vi "Destroy Suite.vi"(8 "error in":errorcluster, 11 "Platano":refnum<class "Platano.CarayaTestSuite.lvclass">) -> (0 "error out":errorcluster, 3 "Test Suite Results":refnum<class "Test Result.lvclass">)   [LabVIEW 2021, in "Banana.Caraya.lvlib" / "Platano.CarayaTestSuite.lvclass"]
uses:
  Platano.CarayaTestSuite.lvclass
  C:/Repositories/LVOS/Bananas/lv-src/Bananas/Platano/Platano.lvclass
  <vilib>/addons/_JKI Toolkits/Caraya/classes/Test Result/Test Result.lvclass
  Bananas/Banana Core Actions -- enum.ctl
  Platano.CarayaTestSuite.lvclass/Platano.CarayaTestSuite.ctl
  Bananas/Banana/Banana.lvclass/Banana.ctl
  <vilib>/LabVIEW Open Source Project/Data Manipulation/Variant/Variant_SetName.vi
  <vilib>/LabVIEW Open Source Project/Data Manipulation/Variant/Variant_BuildClusterFromElementArray.vi
  Bananas/Banana/Read Ephemerals.vi
  <vilib>/LabVIEW Open Source Project/Data Manipulation/Variant/Variant_EmptyCluster.vi
  Leaf.Properties.Suite/Leaf.Properties.Suite.lvclass
  C:/Repositories/LVOS/Bananas/lv-src/Bananas/Leaf.TestSuite/Leaf.TestSuite.lvclass
  Bananas/DestroySuite/DestroySuite.lvclass
  C:/Repositories/LVOS/Bananas/lv-src/Bananas/BananaPeel/BananaPeel.lvclass
  Pips.TestResults/Pips.TestResults.lvclass
  C:/Repositories/LVOS/Bananas/lv-src/Bananas/Pips/Pips.lvclass
  <vilib>/LabVIEW Open Source Project/Data Manipulation/Variant/Variant_ListElements.vi
  <vilib>/LabVIEW Open Source Project/Data Manipulation/TypeDescriptor/TypeDescriptor_SetName.vi
  <vilib>/Utility/GetType.llb/TD_Create Cluster.vi
  Bananas/DefineTest/DefineTest.lvclass
  Bananas/DefineSuite/DefineSuite.lvclass
  Bananas/BananaPeel/BananaPeel.lvclass
  <vilib>/addons/_JKI Toolkits/Caraya/classes/Test Suite/Test Suite.lvclass
  Bananas/Banana/Banana.lvclass
  Bananas/Platano/Platano.lvclass
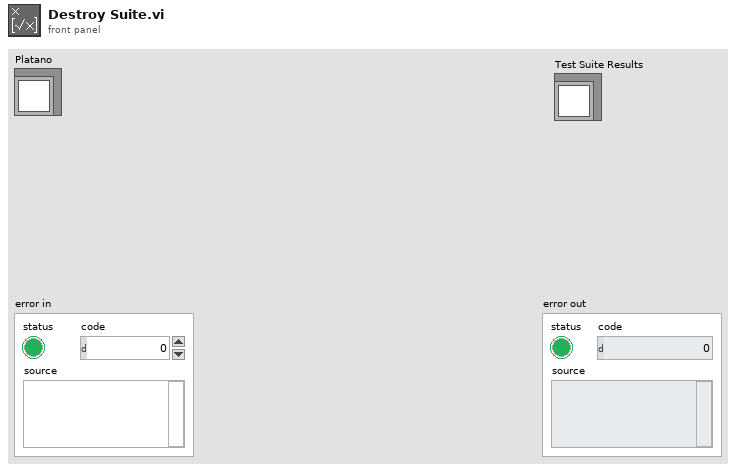
[diagram p1: front panel]
types:
  T1 = typedef "Bananas.lvlib/Banana.lvclass/Banana Core Actions -- enum.ctl" = enum16{"Get/Set", "Clear", "Discard"}
  T2 = typedef "Bananas.lvlib/Test Strategies -- cluster.ctl" = cluster{"DefineTest":refnum<class "DefineTest.lvclass">, "DefineSuite":refnum<class "DefineSuite.lvclass">, "DestroySuite":refnum<class "DestroySuite.lvclass">}
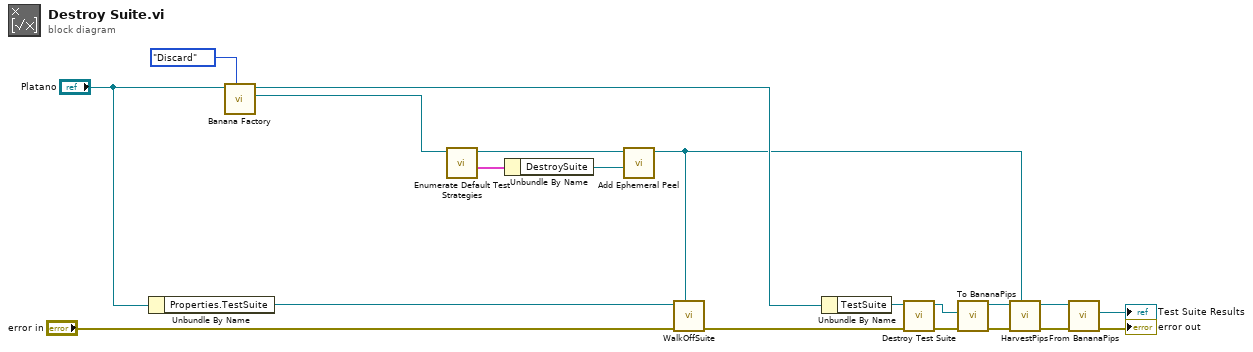
[diagram p0: block diagram]
diagram:
  n1 = Unbundle By Name("Platano") -> ("Properties.TestSuite"=w8:refnum<class "Leaf.Properties.Suite.lvclass">)
  n2 = call "Banana Factory.vi"("Action"=Banana_Core_Actions_--_enum."Discard", "Platano"="Platano") -> ("Banana"=w13:refnum<class "Banana.lvclass">, "Platano dup"=w16:refnum<class "Platano.CarayaTestSuite.lvclass">)  [unwired: 8 in]
  n3 = call "Enumerate Default Test Strategies.vi"("Banana"=w13) -> ("Strategies"=w18:T2, "Banana"=w17:refnum<class "Banana.lvclass">)  [unwired: 9 in]
  n4 = Unbundle By Name(w18) -> ("DestroySuite"=w14:refnum<class "DestroySuite.lvclass">)
  n5 = call "Add Ephemeral Peel.vi"("BananaPeel"=w14, "Banana"=w17) -> ("Banana"=w4:refnum<class "Banana.lvclass">)  [unwired: 9 in]
  n6 = call "WalkOffSuite.vi"("Banana"=w4, "error in (no error)"="error in", "Leaf.TestSuite"=w8) -> ("error out"=w9:errorcluster)  [unwired: 7 in, 1 out]
  n7 = Unbundle By Name(w16) -> ("TestSuite"=w11:refnum<class "Test Suite.lvclass">)
  n8 = call-dynamic "Destroy Test Suite.vi"("error in (no error)"=w9, "Test Suite in"=w11) -> ("error out"=w2:errorcluster, "Test Suite Results"=w7:refnum<class "Test Result.lvclass">)  [unwired: 8 in]
  n9 = call "To BananaPips.vi"("Test Result"=w7) -> ("Pips.TestResults"=w5:refnum<class "Pips.TestResults.lvclass">)  [unwired: 10 in]
  n10 = call "HarvestPips.vi"("Banana"=w4, "error in (no error)"=w2, "Pips"=w5) -> ("error out"=→"error out":errorcluster, "Pips"=w3:refnum<class "Pips.TestResults.lvclass">)  [unwired: 7 in]
  n11 = call "From BananaPips.vi"("Pips.TestResults"=w3) -> ("Test Result"=→"Test Suite Results":refnum<class "Test Result.lvclass">)  [unwired: 10 in]
